vi "VerifyProjectPath.vi"(8 "error in (no error)":errorcluster, 11 "RunUnitTests in":refnum<class "RunUnitTests.lvclass">) -> (0 "error out":errorcluster, 3 "RunUnitTests out":refnum<class "RunUnitTests.lvclass">)   [LabVIEW 2014, in "RunUnitTests.lvclass"]
uses:
  RunUnitTests.lvclass
  RunUnitTests.lvclass/RunUnitTests.ctl
  Utilities/OperationErrorType.ctl
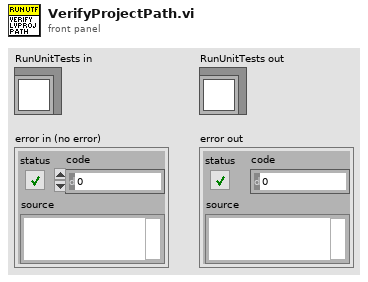
[diagram p1: front panel]
types:
  T1 = typedef "OperationErrorType.ctl" = enum16{"RequiredArgumentMissing", "UnknownArguments", "LoggerSetMultipleTimes", "OperationBrokenError"}
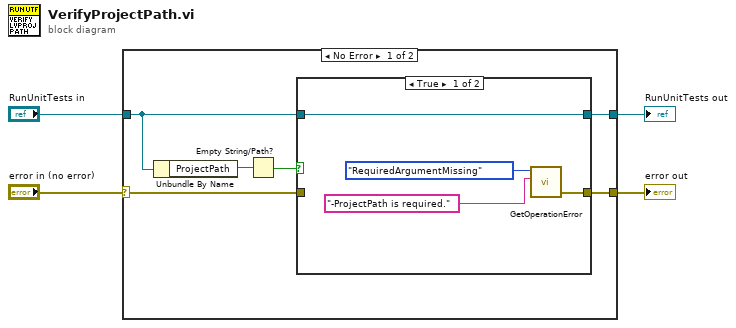
[diagram p0: block diagram]
diagram:
  n1 = case shown="No Error" "error in (no error)" {
    selector: "error in (no error)" -> [w7 w18]
    tunnel: [w10 w18] -> w4
    tunnel: "RunUnitTests in" -> [w9 w17]
    tunnel: [w8 w17] -> w2
    frame No Error {
      n2 = Unbundle By Name(w9) -> ("ProjectPath"=w5:path)
      n3 = Empty String/Path?(string/path=w5) -> (empty?=w6:bool)
      n4 = case shown="True" w6 {
        tunnel: [w14 w16] -> w8
        tunnel: w9 -> [w14 w16]
        tunnel: [w11 w15] -> w10
        tunnel: w7 -> [_ w15]
        frame True {
          n5 = call "GetOperationError.vi"("Additional Information"="-ProjectPath is required.", "Operation Error Type"=OperationErrorType."RequiredArgumentMissing") -> ("error out"=w11:errorcluster)  [unwired: 9 in]
        }
        frame False {
        }
      }
    }
    frame Error {
    }
  }
  "error out" <- w4
  "RunUnitTests out" <- w2
